vi "Stop Haptic Loop.vi"(8 "error in (no error)":errorcluster) -> (0 "error out":errorcluster)   [LabVIEW 2017, in "Haptic Prog Interface.lvlib"]
doc: "Stops the haptic loop, not necessary but ideal for a safe shutdown."
uses:
  Haptic Prog Interface.lvlib
  Haptic-Programming-Interface/src/x64/Debug/Haptic Programming Interface.dll
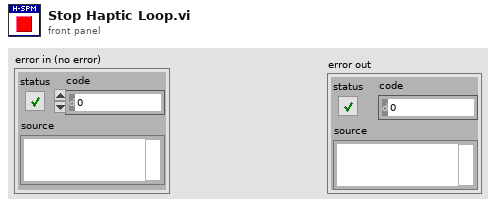
[diagram p1: front panel]
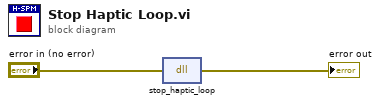
[diagram p0: block diagram]
diagram:
  n1 = dll-call lib="C:/Users/freem/Documents/GitHub/HapticSPM/Haptic-Programming-Interface/src/x64/Debug/Haptic Programming Interface.dll" fn="stop_haptic_loop"(error in="error in (no error)") -> (error out=→"error out":errorcluster)  [unwired: 3 in, 1 out]
